vi "String EQ.vi"(11 "Data In":string) -> (3 "Data Out":string)   [LabVIEW 2016]
uses:
  Core/Assert API Components/Failure Actions.ctl
  Core/Assert API Components/VI References.ctl
  Core/Assert API Components/Assert API Components.lvlib
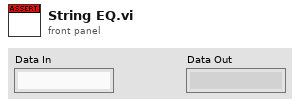
[diagram p1: front panel]
types:
  T1 = typedef "Assert API Components.lvlib/VI References.ctl" = cluster{"Calling VI Ref":refnum<vi>, "Assert VI Ref":refnum<vi>}
  T2 = typedef "Assert API Components.lvlib/Failure Actions.ctl" = enum16{"None", "Log To File", "Pause Execution", "Abort Execution"}
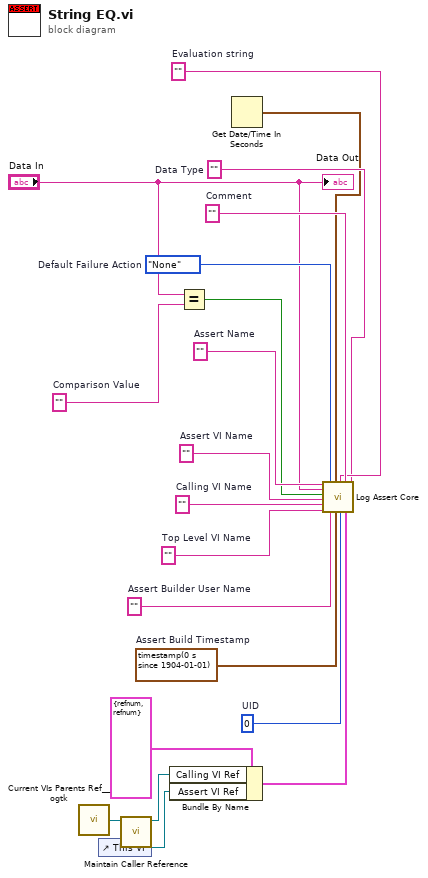
[diagram p0: block diagram]
diagram:
  w2 = ""  # Top Level VI Name
  w4 = 0  # UID
  w5 = ""  # Assert VI Name
  w6 = ""  # Calling VI Name
  w7 = timestamp(0 s since 1904-01-01)  # Assert Build Timestamp
  w8 = ""  # Assert Builder User Name
  w9 = ""  # Data Type
  w17 = ""  # Comment
  w14 = ""  # Evaluation string
  w19 = Failure_Actions."None"  # Default Failure Action
  w20 = ""  # Assert Name
  w18 = ""  # Comparison Value
  n1 = call <userlib>:"Current VIs Parents Ref__ogtk.vi"() -> ("Calling VI's Reference"=w12:refnum<vi>)  [unwired: 2 in]
  n2 = control-ref of="This VI"() -> (w11:refnum<vi>)
  n3 = call "Maintain Caller Reference.vi"("VI in"=w12) -> ("VI out"=w1:refnum<vi>)  [unwired: 10 in]
  n4 = Bundle By Name(cluster=T1 {"Calling VI Ref"=refnum, "Assert VI Ref"=refnum} ("VI References"), "Calling VI Ref"=w1, "Assert VI Ref"=w11) -> (w10:T1)
  n5 = Equal?(x="Data In", y=w18) -> (x = y?=w15:bool)
  n6 = Get Date/Time In Seconds() -> (seconds since 1Jan1904=w3:timestamp)
  n7 = call "Log Assert Core.vi"("Assert Name"=w20, "Data Value"="Data In", "Status"=w15, "Assert VI Name"=w5, "Calling VI Name"=w6, "Top Level VI Name"=w2, "Failure Action"=w19, "Assert Builder User Name"=w8, "Last Update"=w3, "Assert Build Timestamp"=w7, "Evaluation String"=w14, "Assert VI UID"=w4, "Comment"=w17, "VI References"=w10, "Data Type"=w9) -> ()  [unwired: 5 in]
  "Data Out" <- "Data In"
